vi "AuxFindFluo.vi"(6 "camera?":bool, 7 "nruns":i32, 8 "error in (no error)":errorcluster, 11 "READOUT":T1) -> (0 "error out":errorcluster, 3 "av fluo":dbl)   [LabVIEW 2019]
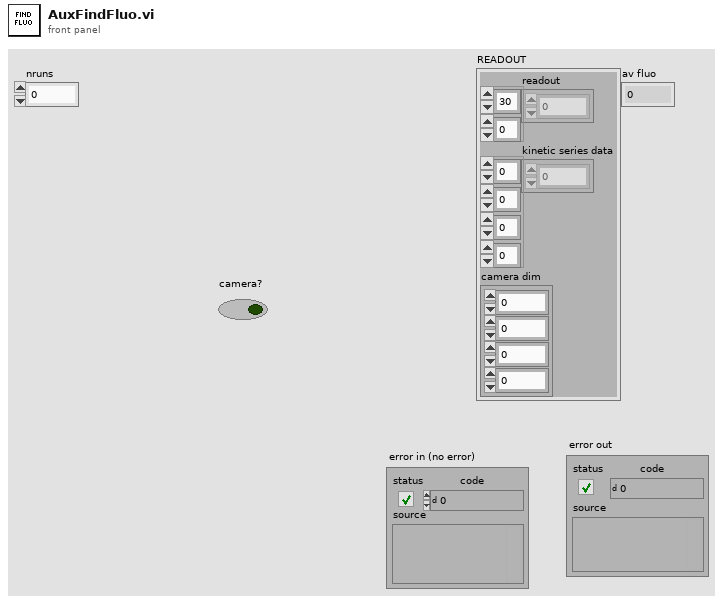
[diagram p1: front panel]
types:
  T1 = cluster{"readout":u32[][], "kinetic series data":i32[][][][], "camera dim":cluster{i32, i32, i32, i32}}
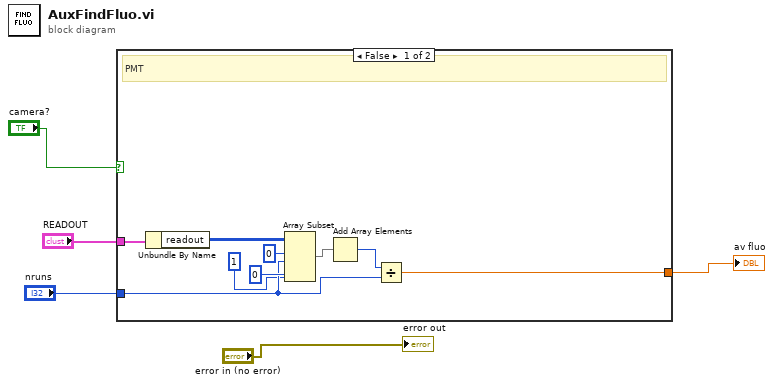
[diagram p0: block diagram]
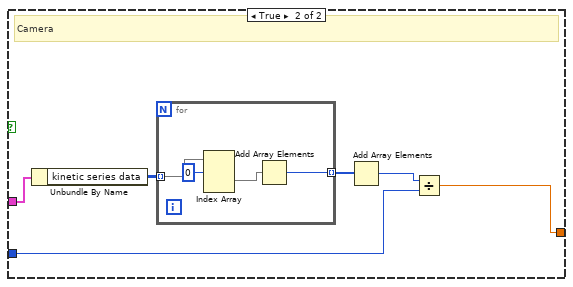
[diagram p2: hidden frame]
diagram:
  n1 = case shown="False" "camera?" {
    tunnel: "READOUT" -> [w14 w20]
    tunnel: "nruns" -> [w7 w16]
    tunnel: [w12 w15] -> w1
    frame False {
      # "PMT"
      n2 = Unbundle By Name(w14) -> ("readout"=w9:u32[][])
      n3 = Array Subset(array=w9, index (row)=0 ("index"), length (row)=w7, index (col)=0 ("index"), length (col)=1 ("length")) -> (w11:u32[][])
      n4 = Add Array Elements(numeric array=w11) -> (sum=w10:u32)
      n5 = Divide(x=w10, y=w7) -> (x/y=w12:dbl)
    }
    frame True {
      # "Camera"
      n6 = Unbundle By Name(w20) -> ("kinetic series data"=w19:i32[][][][])
      n7 = for {
        tunnel: w19 -> [w24] mode=indexing
        tunnel: [w21] -> w18 mode=indexing
        n8 = Index Array(array=w24, index (dim 0)=0 ("index (page)")) -> (element=w22:i32[][])  [unwired: 2 in]
        n9 = Add Array Elements(numeric array=w22) -> (sum=w21:i32)
      }
      n10 = Add Array Elements(numeric array=w18) -> (sum=w17:i32)
      n11 = Divide(x=w17, y=w16) -> (x/y=w15:dbl)
    }
  }
  "av fluo" <- w1
  "error out" <- "error in (no error)"
